vi "Set Connection ID.vi"(11 "TCP Network Connection in":refnum<k5>) -> (3 "connection info out":T1)   [LabVIEW 2016, in "Assert Service.lvlib" / "Assert Service.lvclass"]
uses:
  Assert Service.lvclass
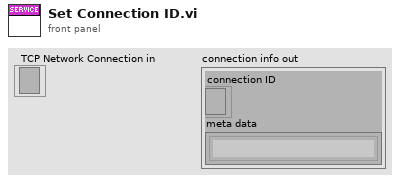
[diagram p1: front panel]
types:
  T1 = cluster{"connection ID":refnum<k5>, "meta data":string[]}
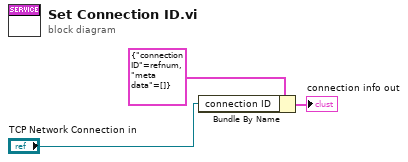
[diagram p0: block diagram]
diagram:
  n1 = Bundle By Name(cluster=T1 {"connection ID"=refnum, "meta data"=[]} ("connection info out"), "connection ID"="TCP Network Connection in") -> (→"connection info out":T1)
